vi "Build Query String.vi"(4 "Query Map":map{string, string}(c390)) -> (7 "Query String":string)   [LabVIEW 2020, in "URI.lvlib"]
uses:
  URI.lvlib
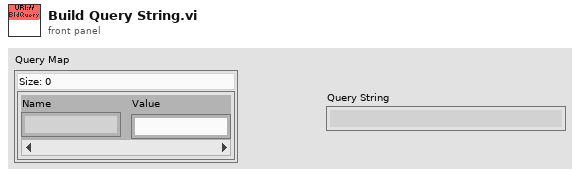
[diagram p1: front panel]
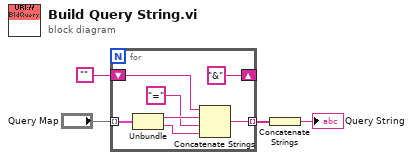
[diagram p0: block diagram]
diagram:
  n1 = for {
    tunnel: "Query Map" -> [w11] mode=indexing
    shift-right: ["&"] -> _
    shift-left: "" -> [w7]
    tunnel: [w5] -> w2 mode=indexing
    n2 = Unbundle(w11) -> ("Name"=w10:string, "Value"=w9:string)
    n3 = Concatenate Strings(w7, w10, "=", w9) -> (w5:string)
  }
  n4 = Concatenate Strings(w2) -> (→"Query String":string)
